vi "DK240 SlitInfo.vi"(5 "Port":refnum<visa-resource-name>="SPECTRO", 7 "error in":errorcluster) -> (0 "S1 width":u16 caption="Fente 1 (µm)" max=5000 step=1, 1 "S2 width":u16 caption="Fente 2 (µm)" max=5000 step=1, 2 "Status":u8, 3 "error out":errorcluster)   [LabVIEW 2019]
doc: "Ce VI retourne la largeurs actuelle des fentes.\n\nThis VI returns the current slit widths."
uses:
  <vilib>/Utility/error.llb/DialogType.ctl
panel:
  out "Cancel":u8
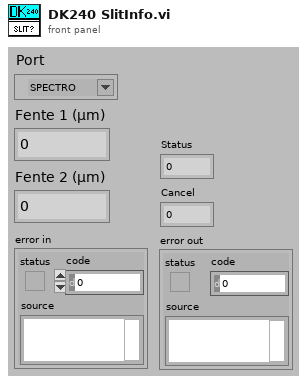
[diagram p1: front panel]
types:
  T1 = typedef "DialogType.ctl" = u16
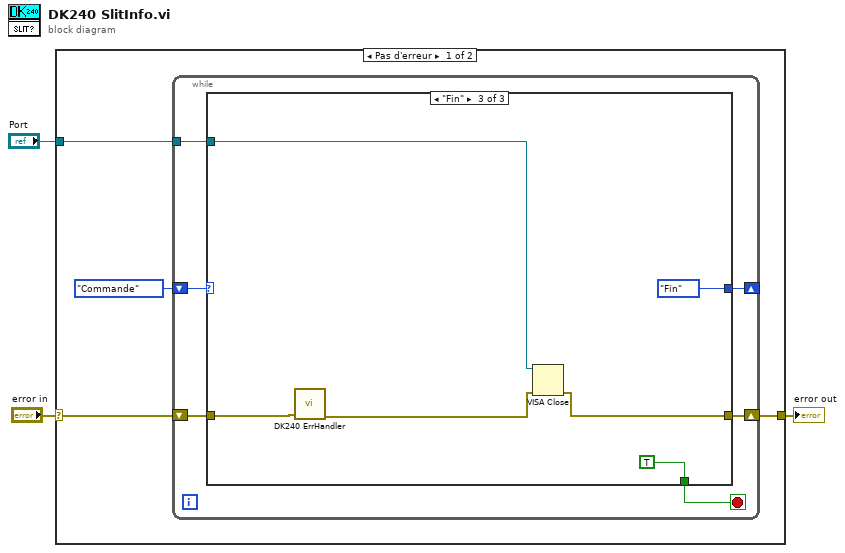
[diagram p0: block diagram]
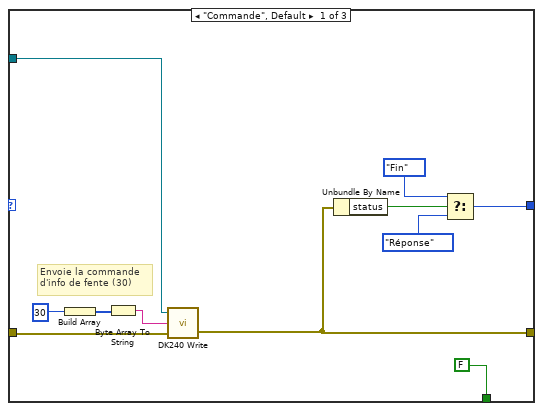
[diagram p2: hidden frame]
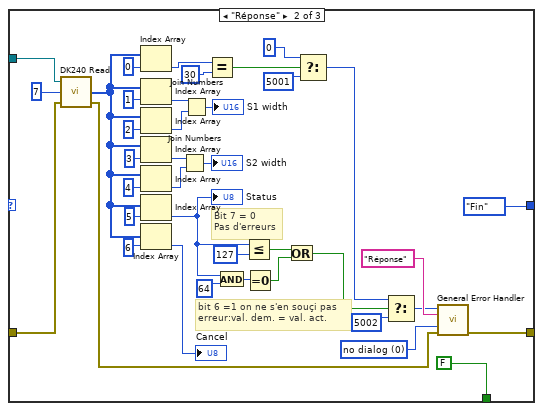
[diagram p3: hidden frame]
diagram:
  n1 = case shown="Pas d'erreur" "error in" {
    selector: "error in" -> [w4 w70]
    tunnel: "Port" -> [w7 _]
    tunnel: [w6 w70] -> w2
    frame No Error {
      n2 = while {
        tunnel: w7 -> [w12]
        shift-right: [w10] -> w6
        shift-left: w4 -> [w11]
        shift-right: [w8] -> _
        shift-left: enum16{"Commande", "Réponse", "Fin"}."Commande" -> [w9]
        stop <- w13 stop-if-true
        n3 = case shown="\"Fin\"" w9 {
          tunnel: [FALSE FALSE TRUE] -> w13
          tunnel: w12 -> [w20 w52 w66]
          tunnel: w11 -> [w19 w51 w65]
          tunnel: [w16 w36 w67] -> w10
          tunnel: [w14 enum16{"Commande", "Réponse", "Fin"}."Fin" enum16{"Commande", "Réponse", "Fin"}."Fin"] -> w8
          frame "Commande", Default {
            # "Envoie la commande\nd'info de fente (30)"
            n4 = Build Array(u8 30) -> (w24:u8[])
            n5 = Byte Array To String(unsigned byte array=w24) -> (string=w21:string)
            n6 = call <userlib>:"DK240 Write.vi"("error in"=w19, "String to write"=w21, "Port"=w20) -> ("error out"=w16:errorcluster)  [unwired: 1 in]
            n7 = Unbundle By Name(w16) -> ("status"=w15:bool)
            n8 = Select(t=enum16{"Commande", "Réponse", "Fin"}."Fin", s=w15, f=enum16{"Commande", "Réponse", "Fin"}."Réponse") -> (s? t:f=w14:enum16{"Commande", "Réponse", "Fin"})
          }
          frame "Réponse" {
            w42 = T1 0 items=["no dialog", "OK message", "continue or stop message", "OK message + warnings", "continue/stop + warnings"] ("type of dialog (OK msg:1)")
            # "bit 6 =1 on ne s'en souçi pas \nerreur:val. dem. = val. act."
            # "Bit 7 = 0\nPas d'erreurs"
            n9 = call <userlib>:"DK240 Read.vi"("error in"=w51, "Byte count"=u32 7, "Port"=w52) -> ("error out"=w37:errorcluster, "Received Bytes"=w33:u8[])  [unwired: 1 in]
            n10 = Index Array(array=w33, index=0) -> (element=w29:u8)
            n11 = Index Array(array=w33, index=1) -> (element=w57:u8)
            n12 = Index Array(array=w33, index=2) -> (element=w56:u8)
            n13 = Index Array(array=w33, index=3) -> (element=w55:u8)
            n14 = Index Array(array=w33, index=4) -> (element=w54:u8)
            n15 = Index Array(array=w33, index=5) -> (element=w25:u8)
            "Status" <- w25
            n16 = Index Array(array=w33, index=6) -> (element=→"Cancel":u8)
            n17 = Join Numbers(hi=w55, lo=w54) -> ((hi.lo)=→"S2 width":u16)
            n18 = Join Numbers(hi=w57, lo=w56) -> ((hi.lo)=→"S1 width":u16)
            n19 = Equal?(x=w29, y=u8 30) -> (x = y?=w27:bool)
            n20 = And(x=w25, y=u8 64) -> (x .and. y?=w44:u8)
            n21 = Less Or Equal?(x=w25, y=u8 127) -> (x <= y?=w45:bool)
            n22 = Equal To 0?(x=w44) -> (x = 0?=w46:bool)
            n23 = Or(x=w45, y=w46) -> (x .or. y?=w47:bool)
            n24 = Select(t=0, s=w27, f=5001 ("t")) -> (s? t:f=w26:i32)
            n25 = Select(t=w26, s=w47, f=5002 ("t")) -> (s? t:f=w39:i32)
            n26 = call <vilib>:"General Error Handler.vi"("[error code] (0)"=w39, "[error source] (\" \")"="Réponse" ("[error source] (\" \")"), "type of dialog (OK msg:1)"=w42, "error in (no error)"=w37) -> ("error out"=w36:errorcluster)  [unwired: 7 in, 4 out]
          }
          frame "Fin" {
            n27 = call <userlib>:"DK240 ErrHandler.vi"("error in"=w65) -> ("error out"=w64:errorcluster)  [unwired: 7 in]
            n28 = VISA Close(VISA resource name=w66, error in (no error)=w64) -> (error out=w67:errorcluster)
          }
        }
      }
    }
    frame Error {
    }
  }
  "error out" <- w2
